vi "Do_Every_minute.vi"(1 "Ch Names":string[](array[string]), 2 "Values":dbl[](array[numeric]) format="%.2f") -> ()   [LabVIEW 2012]
uses:
  Do_Every_5mins.ctl
  Anemometry/Anemometry Sub Vis/Controls/In_Range.ctl
  ADAM Client/Sub VIs/ADAM Controls/Traverse_Level_State.ctl
  ADAM Client/Sub VIs/ADAM Controls/Valco_valve_ph.ctl
  ADAM_Global.vi
panel:
  in  "Disable Sending email to estates regarding Chilled water Temp":bool=TRUE
  in  "Max K Factor":dbl=2.7
  out "Case":T1
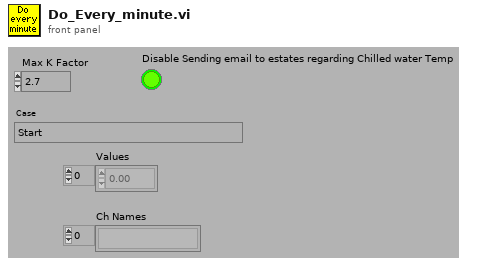
[diagram p1: front panel]
types:
  T1 = typedef "Do_Every_5mins.ctl" = enum16{"Start", "Update EnFlo Tunnel Speed Tweak", "Are EnFlo Tun Fan Bearings too Hot?", "Check EnFlo tweak factor?", "Are Inlet Screens Blocked?", "Tweak demanded chilled water temp", "Is Dew point meter Alive?", "Condensation Occurring", "Condensation Alert", "More checks", "Set FFID Valve to Measure", "End"}
  T2 = typedef "In_Range.ctl" = enum16{"%", "±", "% & ±"}
  T3 = typedef "Traverse_Level_State.ctl" = enum16{"Running", "Complete"}
  T4 = typedef "Client_State_Cluster.ctl" = cluster{"Client Name":string, "Traverse level State":T3, "People to Email":string[], "Next Contact Time":dbl}
  T5 = typedef "Valco_valve_ph.ctl" = u16
  T6 = cluster{"second":i32, "minute":i32, "hour":i32, "day of month":i32, "month":i32, "year":i32, "day of week":i32, "day of year":i32, "is DST":i32}
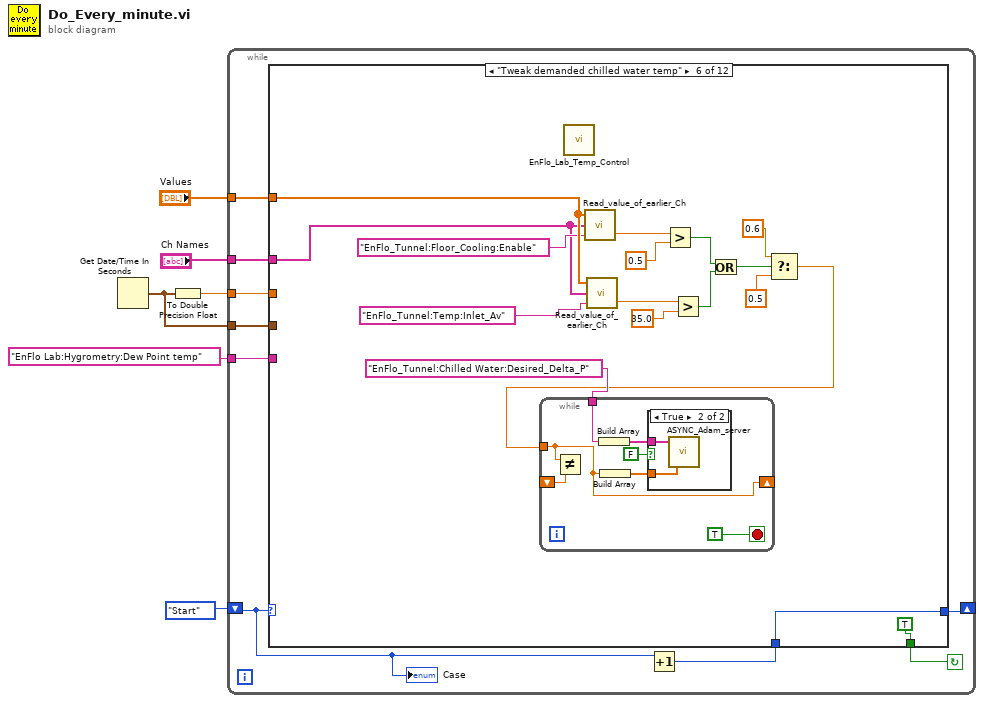
[diagram p0: block diagram]
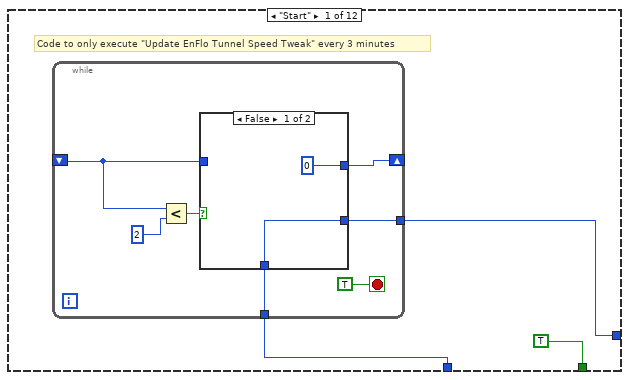
[diagram p2: hidden frame]
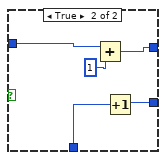
[diagram p3: hidden frame]
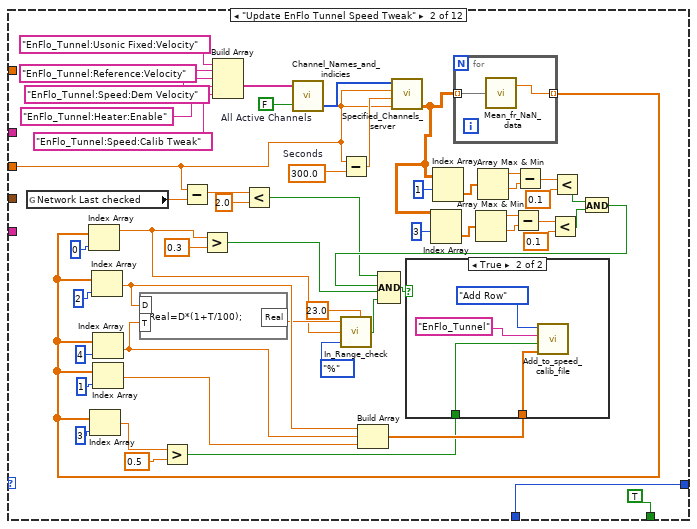
[diagram p4: hidden frame]
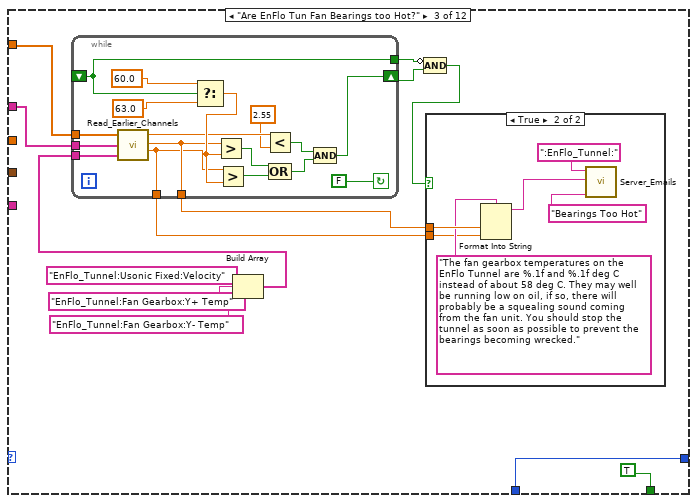
[diagram p6: hidden frame]
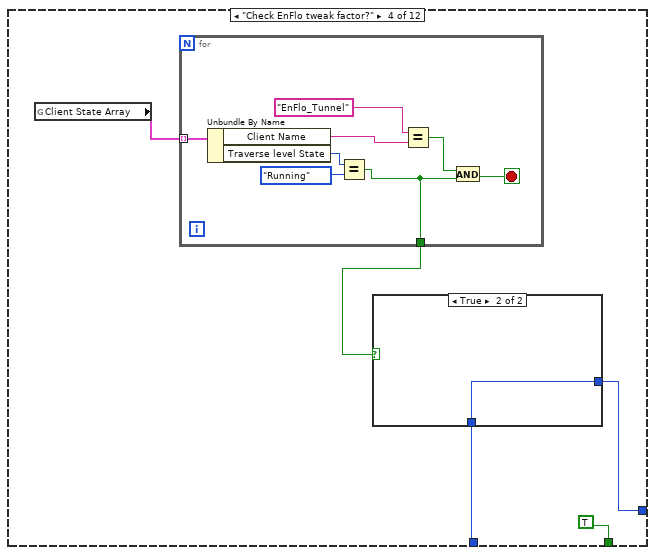
[diagram p8: hidden frame]
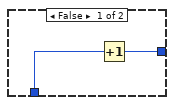
[diagram p9: hidden frame]
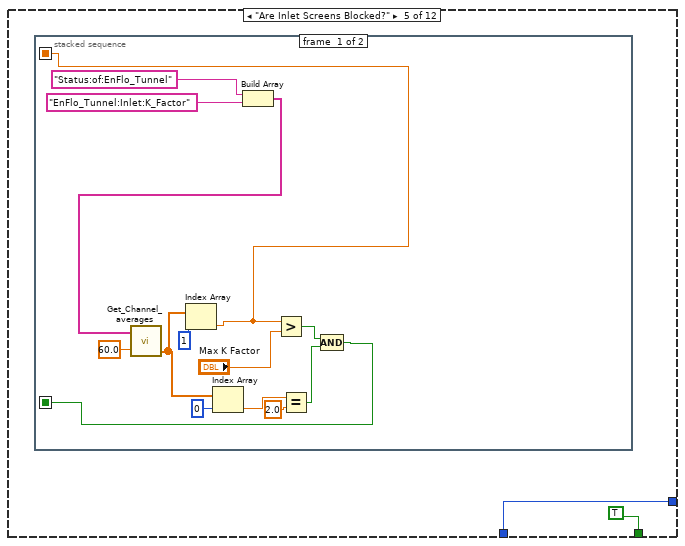
[diagram p10: hidden frame]
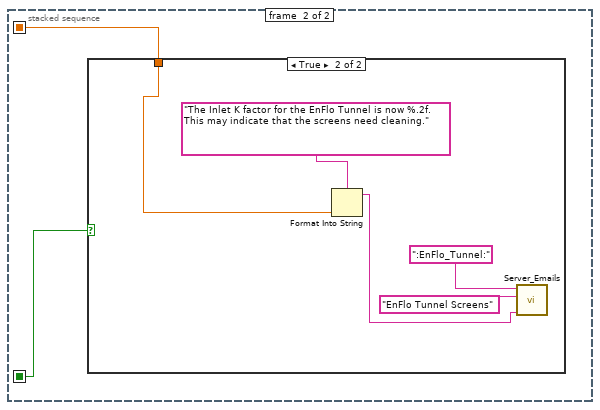
[diagram p11: hidden frame]
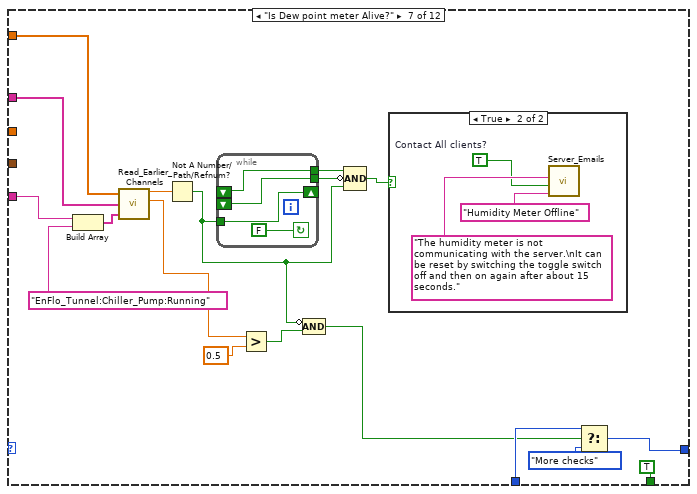
[diagram p14: hidden frame]
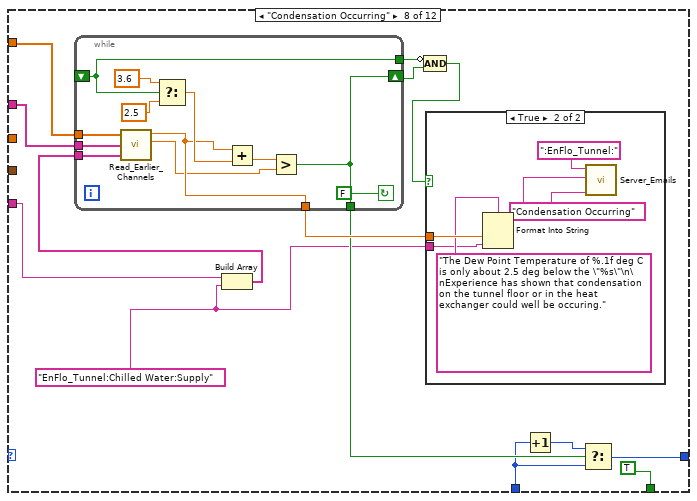
[diagram p16: hidden frame]
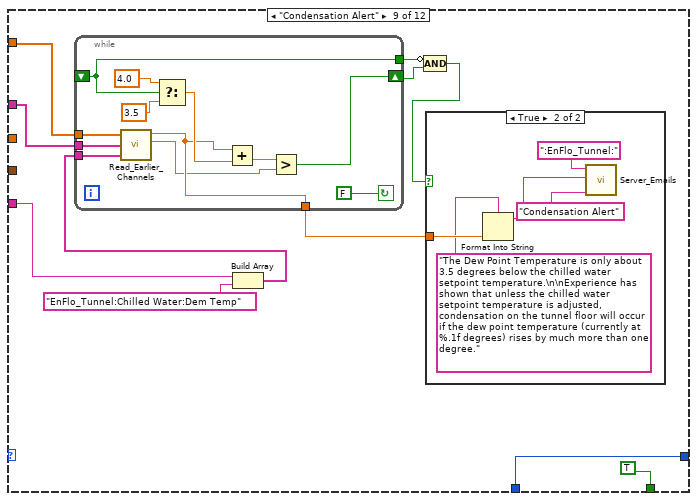
[diagram p18: hidden frame]
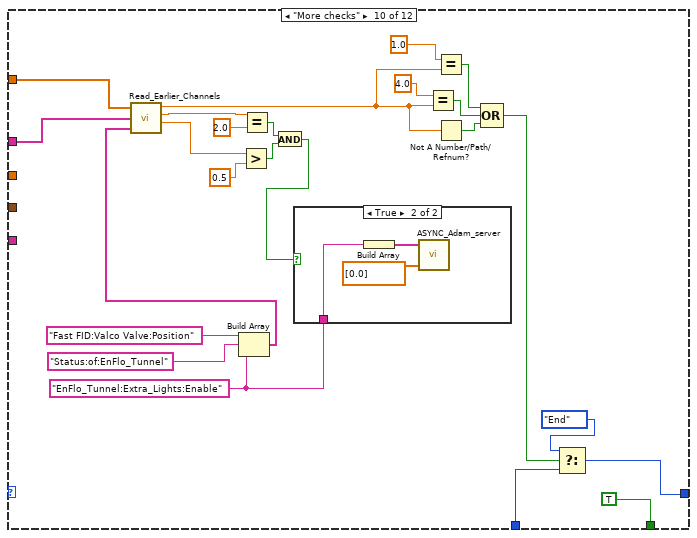
[diagram p20: hidden frame]
diagram:
  n1 = Get Date/Time In Seconds() -> (seconds since 1Jan1904=w1:timestamp)
  n2 = To Double Precision Float(number=w1) -> (double precision float=w2:dbl)
  n3 = while {
    tunnel: "EnFlo Lab:Hygrometry:Dew Point temp" -> [w9]
    tunnel: "Values" -> [w13]
    tunnel: "Ch Names" -> [w14]
    shift-left: Do_Every_5mins."Start" ("Case") -> [w10]
    shift-right: [w11] -> _
    tunnel: w2 -> [w8]
    tunnel: w1 -> [w7]
    stop <- w15 continue-if-true
    n4 = Increment(x=w10) -> (x+1=w12:T1)
    n5 = case shown="\"Tweak demanded chilled water temp\"" w10 {
      tunnel: [TRUE TRUE TRUE TRUE TRUE TRUE TRUE TRUE TRUE TRUE TRUE FALSE] -> w15
      tunnel: w14 -> [_ _ w102 _ _ w179 w207 w230 w257 w300 w307 w340]
      tunnel: w13 -> [_ _ w103 _ _ w181 w208 w231 w258 w301 w306 w339]
      tunnel: w12 -> [w16 w74 w93 w131 w145 w184 w199 w221 w260 w298 w325 w343]
      tunnel: [w17 w74 w93 w130 w145 w184 w211 w222 w260 w297 w325 w343] -> w11
      tunnel: w9 -> [_ _ _ _ _ _ w206 w224 w251 _ _ _]
      tunnel: w8 -> [_ w34 _ _ _ _ _ _ _ _ w324 _]
      tunnel: w7 -> [_ _ _ _ _ _ _ _ _ _ _ w341]
      frame "Start" {
        # "Code to only execute \"Update EnFlo Tunnel Speed Tweak\" every 3 minutes"
        n6 = while {
          shift-right: [w22] -> _
          shift-left: _ -> [w19]
          tunnel: [w21] -> w17
          tunnel: w16 -> [w20]
          stop <- TRUE stop-if-true
          n7 = Less?(x=w19, y=2) -> (x < y?=w23:bool)
          n8 = case shown="False" w23 {
            tunnel: [0 w30] -> w22
            tunnel: [w26 w28] -> w21
            tunnel: w20 -> [w26 w29]
            tunnel: w19 -> [_ w31]
            frame False {
            }
            frame True {
              n9 = Add(x=w31, y=1) -> (x+y=w30:i32)
              n10 = Increment(x=w29) -> (x+1=w28:T1)
            }
          }
        }
      }
      frame "Update EnFlo Tunnel Speed Tweak" {
        w68 = 300.0  # Seconds
        w70 = FALSE  # All Active Channels
        n11 = global read "ADAM_Global.vi" "Network Last checked"() -> (w35:dbl)
        n12 = Subtract(x=w34, y=w35) -> (x-y=w36:dbl)
        n13 = Build Array("EnFlo_Tunnel:Usonic Fixed:Velocity", "EnFlo_Tunnel:Reference:Velocity", "EnFlo_Tunnel:Speed:Dem Velocity", "EnFlo_Tunnel:Heater:Enable", "EnFlo_Tunnel:Speed:Calib Tweak") -> (w67:string[])
        n14 = Less?(x=w36, y=2.0) -> (x < y?=w33:bool)
        n15 = call "Channel_Names_and_indicies.vi"("All Active Channels"=w70, "Desired Ch Names"=w67) -> ("Indicies"=w69:i32[])  [unwired: 1 out]
        n16 = Subtract(x=w34, y=w68) -> (x-y=w66:dbl)
        n17 = call "Specified_Channels_server.vi"("End time"=w34, "Start time"=w66, "Clients time"=w34, "Requested channels"=w69) -> ("Output array"=w48:dbl[][])  [unwired: 1 in, 4 out]
        n18 = Index Array(array=w48, index (row)=3 ("Index")) -> (element=w50:dbl[])  [unwired: 1 in]
        n19 = Index Array(array=w48, index (row)=1 ("Index")) -> (element=w64:dbl[])  [unwired: 1 in]
        n20 = for {
          tunnel: w48 -> [w88] mode=indexing
          tunnel: [w87] -> w57 mode=indexing
          n21 = call "Mean_fr_NaN_data.vi"("Data"=w88) -> ("Mean value"=w87:dbl)  [unwired: 1 out]
        }
        n22 = Index Array(array=w57, index=0) -> (element=w41:dbl)
        n23 = Index Array(array=w57, index=3) -> (element=w77:dbl)
        n24 = Index Array(array=w57, index=2) -> (element=w43:dbl)
        n25 = Index Array(array=w57, index=4) -> (element=w44:dbl)
        n26 = Index Array(array=w57, index=1) -> (element=w55:dbl)
        n27 = formula code="Real=D*(1+T/100);"("D"=w43, "T"=w44) -> ("Real"=w42:dbl)
        n28 = Greater?(x=w77, y=0.5) -> (0:w56:bool)
        n29 = Greater?(x=w41, y=0.3) -> (0:w75:bool)
        n30 = call "In_Range_check.vi"("%"=23.0, "Mode"=In_Range."%", "Value"=w41, "Setpoint"=w42) -> ("In Range"=w38:bool)  [unwired: 1 in, 2 out]
        n31 = Build Array(w43, w44, w55) -> (w72:dbl[])
        n32 = Array Max & Min(array=w50) -> (max value=w51:dbl, min value=w52:dbl)  [unwired: 2 out]
        n33 = Array Max & Min(array=w64) -> (max value=w63:dbl, min value=w62:dbl)  [unwired: 2 out]
        n34 = Subtract(x=w51, y=w52) -> (x-y=w53:dbl)
        n35 = Subtract(x=w63, y=w62) -> (x-y=w61:dbl)
        n36 = Less?(x=w53, y=0.1) -> (x < y?=w47:bool)
        n37 = Less?(x=w61, y=0.1) -> (x < y?=w46:bool)
        n38 = And(x=w46, y=w47) -> (x .and. y?=w45:bool)
        n39 = Compound Arithmetic op=AND(w33, w45, w75, w38) -> (w71:bool)
        n40 = case shown="True" w71 {
          tunnel: w72 -> [_ w91]
          tunnel: w56 -> [_ w90]
          frame False {
          }
          frame True {
            n41 = call "Add_to_speed_calib_file.vi"("New Row"=w91, "Tunnel Heated?"=w90, "Rig Name"="EnFlo_Tunnel" ("y"), "Mode"=enum16{"Add Row", "Get Error Value"}."Add Row") -> ()  [unwired: 2 in, 2 out]
          }
        }
      }
      frame "Are EnFlo Tun Fan Bearings too Hot?" {
        n42 = Build Array("EnFlo_Tunnel:Usonic Fixed:Velocity", "EnFlo_Tunnel:Fan Gearbox:Y+ Temp", "EnFlo_Tunnel:Fan Gearbox:Y- Temp") -> (w101:string[])
        n43 = while {
          tunnel: [w107] -> w94
          tunnel: [w108] -> w95
          tunnel: [w117] -> w100
          shift-left: _ -> [w117]
          shift-right: [w109] -> w99
          tunnel: w101 -> [w120]
          tunnel: w102 -> [w121]
          tunnel: w103 -> [w122]
          stop <- FALSE continue-if-true
          n44 = call "Read_Earlier_Channels.vi"("Present scan array"=w122, "Ch names"=w121, "Desired Channels"=w120) -> ("Index 0"=w115:dbl, "Index 1"=w108:dbl, "Index 2"=w107:dbl)  [unwired: 3 out]
          n45 = Select(t=60.0, s=w117, f=63.0) -> (s? t:f=w116:dbl)
          n46 = Greater?(x=w108, y=w116) -> (0:w113:bool)
          n47 = Greater?(x=w107, y=w116) -> (0:w112:bool)
          n48 = Less?(x=w115, y=2.55) -> (x < y?=w111:bool)
          n49 = Compound Arithmetic op=OR(w113, w112) -> (w110:bool)
          n50 = Compound Arithmetic op=AND(w111, w110) -> (w109:bool)
        }
        n51 = Compound Arithmetic op=AND(invert w100, w99) -> (w98:bool)
        n52 = case shown="True" w98 {
          tunnel: w95 -> [_ w126]
          tunnel: w94 -> [_ w123]
          frame False {
          }
          frame True {
            n53 = Format Into String(format string="The fan gearbox temperatures on the EnFlo Tunnel are %.1f and %.1f deg C instead of about 58 deg C. They may well be running low on oil, if so, there will probably be a squealing sound coming from the fan unit. You should stop the tunnel as soon as possible to prevent the bearings becoming wrecked." ("Format String"), w126, w123) -> (resulting string=w125:string)  [unwired: 2 in, 1 out]
            n54 = call "Server_Emails.vi"("Client Name Contains"=":EnFlo_Tunnel:", "Message"=w125, "Subject"="Bearings Too Hot" ("Error Type")) -> ()  [unwired: 2 in, 3 out]
          }
        }
      }
      frame "Check EnFlo tweak factor?" {
        n55 = global read "ADAM_Global.vi" "Client State Array"() -> (w132:T4[])
        n56 = for {
          tunnel: w132 -> [w144] mode=indexing
          tunnel: [w137] -> w129
          stop <- w138 stop-if-true
          n57 = Unbundle By Name(w144) -> ("Client Name"=w140:string, "Traverse level State"=w143:T3)
          n58 = Equal?(x=w143, y=Traverse_Level_State."Running" ("Traverse level State")) -> (x = y?=w137:bool)
          n59 = Equal?(x="EnFlo_Tunnel" ("y"), y=w140) -> (x = y?=w139:bool)
          n60 = And(x=w139, y=w137) -> (x .and. y?=w138:bool)
        }
        n61 = case shown="True" w129 {
          tunnel: w131 -> [w135 w136]
          tunnel: [w134 w136] -> w130
          frame False {
            n62 = Increment(x=w135) -> (x+1=w134:T1)
          }
          frame True {
          }
        }
      }
      frame "Are Inlet Screens Blocked?" {
        n63 = stacked-sequence {
          seq-local: [w147 _] -> [_ w162]
          seq-local: [w150 _] -> [_ w161]
          frame #0 {
            n64 = Build Array("Status:of:EnFlo_Tunnel", "EnFlo_Tunnel:Inlet:K_Factor") -> (w152:string[])
            n65 = call "Get_Channel_averages.vi"("Desired Ch Names"=w152, "Averaging time (mins)"=60.0) -> ("number"=w158:dbl[])  [unwired: 1 in, 2 out]
            n66 = Index Array(array=w158, index=1) -> (element=w147:dbl)
            n67 = Index Array(array=w158, index=0) -> (element=w157:dbl)
            n68 = Greater?(x=w147, y="Max K Factor") -> (0:w149:bool)
            n69 = Equal?(x=w157, y=2.0) -> (x = y?=w155:bool)
            n70 = Compound Arithmetic op=AND(w149, w155) -> (w150:bool)
          }
          frame #1 {
            n71 = case shown="True" w161 {
              tunnel: w162 -> [_ w166]
              frame False {
              }
              frame True {
                n72 = Format Into String(format string="The Inlet K factor for the EnFlo Tunnel is now %.2f. This may indicate that the screens need cleaning." ("Format String"), w166) -> (resulting string=w164:string)  [unwired: 2 in, 1 out]
                n73 = call "Server_Emails.vi"("Client Name Contains"=":EnFlo_Tunnel:", "Message"="EnFlo Tunnel Screens", "Subject"=w164) -> ()  [unwired: 2 in, 3 out]
              }
            }
          }
        }
      }
      frame "Tweak demanded chilled water temp" {
        n74 = call "EnFlo_Lab_Temp_Control.vi"() -> ()  [unwired: 1 out]
        n75 = call "Read_value_of_earlier_Ch.vi"("Desired Ch to Read"="EnFlo_Tunnel:Floor_Cooling:Enable", "Ch names"=w179, "Present scan array"=w181) -> ("Value"=w177:dbl)  [unwired: 1 in, 1 out]
        n76 = call "Read_value_of_earlier_Ch.vi"("Desired Ch to Read"="EnFlo_Tunnel:Temp:Inlet_Av", "Ch names"=w179, "Present scan array"=w181) -> ("Value"=w175:dbl)  [unwired: 1 in, 1 out]
        n77 = Greater?(x=w177, y=0.5) -> (0:w173:bool)
        n78 = Greater?(x=w175, y=35.0) -> (0:w172:bool)
        n79 = Or(x=w173, y=w172) -> (x .or. y?=w171:bool)
        n80 = Select(t=0.6, s=w171, f=0.5 ("t")) -> (s? t:f=w168:dbl)
        n81 = while {
          shift-right: [w187] -> _
          shift-left: _ -> [w188]
          tunnel: w168 -> [w187]
          tunnel: "EnFlo_Tunnel:Chilled Water:Desired_Delta_P" -> [w189]
          stop <- TRUE stop-if-true
          n82 = Not Equal?(x=w187, y=w188) -> ()  [unwired: 1 out]
          n83 = Build Array(w189) -> (w190:string[])
          n84 = Build Array(w187) -> (w191:dbl[])
          n85 = case shown="True" FALSE {
            tunnel: w191 -> [_ w193]
            tunnel: w190 -> [_ w192]
            frame False {
            }
            frame True {
              n86 = call "ASYNC_Adam_server.vi"("Values"=w193, "Channel Names"=w192) -> ()  [unwired: 1 in, 3 out]
            }
          }
        }
      }
      frame "Is Dew point meter Alive?" {
        n87 = Build Array(w206, "EnFlo_Tunnel:Chiller_Pump:Running") -> (w204:string[])
        n88 = call "Read_Earlier_Channels.vi"("Present scan array"=w208, "Ch names"=w207, "Desired Channels"=w204) -> ("Index 0"=w203:dbl, "Index 1"=w201:dbl)  [unwired: 4 out]
        n89 = Not A Number/Path/Refnum?(number/path/refnum=w203) -> (NaN/Path/Refnum?=w196:bool)
        n90 = while {
          tunnel: [w213] -> w194
          tunnel: [w214] -> w195
          shift-left: _ -> [w214]
          tunnel: w196 -> [w215]
          shift-left: _ -> [w213]
          shift-right: [w215] -> _
          stop <- FALSE continue-if-true
        }
        n91 = Greater?(x=w201, y=0.5) -> (0:w200:bool)
        n92 = Compound Arithmetic op=AND(invert w196, w200) -> (w197:bool)
        n93 = Compound Arithmetic op=AND(w194, invert w195, w196) -> (w209:bool)
        n94 = case shown="True" w209 {
          frame False {
          }
          frame True {
            w216 = TRUE  # Contact All clients?
            n95 = call "Server_Emails.vi"("Message"="The humidity meter is not communicating with the server.\nIt can be reset by switching the toggle switch off and then on again after about 15 seconds." ("Bundle Element"), "Contact All clients?"=w216, "Subject"="Humidity Meter Offline" ("Error Type")) -> ()  [unwired: 2 in, 3 out]
          }
        }
        n96 = Select(t=w199, s=w197, f=Do_Every_5mins."More checks" ("Case")) -> (s? t:f=w211:T1)
      }
      frame "Condensation Occurring" {
        w219 = "EnFlo_Tunnel:Chilled Water:Supply"
        n97 = Build Array(w224, w219) -> (w229:string[])
        n98 = while {
          tunnel: [w234] -> w223
          tunnel: [w236] -> w225
          tunnel: [w237] -> w228
          shift-left: _ -> [w237]
          shift-right: [w234] -> w227
          tunnel: w229 -> [w242]
          tunnel: w230 -> [w243]
          tunnel: w231 -> [w244]
          stop <- FALSE continue-if-true
          n99 = call "Read_Earlier_Channels.vi"("Present scan array"=w244, "Ch names"=w243, "Desired Channels"=w242) -> ("Index 0"=w236:dbl, "Index 1"=w235:dbl)  [unwired: 4 out]
          n100 = Select(t=3.6, s=w237, f=2.5) -> (s? t:f=w238:dbl)
          n101 = Add(x=w236, y=w238) -> (x+y=w241:dbl)
          n102 = Greater?(x=w241, y=w235) -> (0:w234:bool)
        }
        n103 = Compound Arithmetic op=AND(invert w228, w227) -> (w226:bool)
        n104 = case shown="True" w226 {
          tunnel: w225 -> [_ w248]
          tunnel: w219 -> [_ w245]
          frame False {
          }
          frame True {
            n105 = Format Into String(format string="The Dew Point Temperature of %.1f deg C is only about 2.5 deg below the \"%s\"\n\nExperience has shown that condensation on the tunnel floor or in the heat exchanger could well be occuring." ("Format String"), w248, w245) -> (resulting string=w247:string)  [unwired: 2 in, 1 out]
            n106 = call "Server_Emails.vi"("Client Name Contains"=":EnFlo_Tunnel:", "Message"=w247, "Subject"="Condensation Occurring" ("Error Type")) -> ()  [unwired: 2 in, 3 out]
          }
        }
        n107 = Increment(x=w221) -> (x+1=w220:T1)
        n108 = Select(t=w220, s=w223, f=w221) -> (s? t:f=w222:T1)
      }
      frame "Condensation Alert" {
        n109 = Build Array(w251, "EnFlo_Tunnel:Chilled Water:Dem Temp") -> (w256:string[])
        n110 = while {
          tunnel: [w264] -> w252
          tunnel: [w266] -> w255
          shift-left: _ -> [w266]
          shift-right: [w265] -> w254
          tunnel: w256 -> [w271]
          tunnel: w257 -> [w272]
          tunnel: w258 -> [w273]
          stop <- FALSE continue-if-true
          n111 = call "Read_Earlier_Channels.vi"("Present scan array"=w273, "Ch names"=w272, "Desired Channels"=w271) -> ("Index 0"=w264:dbl, "Index 1"=w263:dbl)  [unwired: 4 out]
          n112 = Select(t=4.0, s=w266, f=3.5) -> (s? t:f=w267:dbl)
          n113 = Add(x=w264, y=w267) -> (x+y=w270:dbl)
          n114 = Greater?(x=w270, y=w263) -> (0:w265:bool)
        }
        n115 = Compound Arithmetic op=AND(invert w255, w254) -> (w253:bool)
        n116 = case shown="True" w253 {
          tunnel: w252 -> [_ w276]
          frame False {
          }
          frame True {
            n117 = Format Into String(format string="The Dew Point Temperature is only about 3.5 degrees below the chilled water setpoint temperature.\n\nExperience has shown that unless the chilled water setpoint temperature is adjusted, condensation on the tunnel floor will occur if the dew point temperature (currently at %.1f degrees) rises by much more than one degree." ("Format String"), w276) -> (resulting string=w275:string)  [unwired: 2 in, 1 out]
            n118 = call "Server_Emails.vi"("Client Name Contains"=":EnFlo_Tunnel:", "Message"=w275, "Subject"="Condensation Alert" ("Error Type")) -> ()  [unwired: 2 in, 3 out]
          }
        }
      }
      frame "More checks" {
        w280 = "EnFlo_Tunnel:Extra_Lights:Enable"
        n119 = Build Array("Fast FID:Valco Valve:Position", "Status:of:EnFlo_Tunnel", w280) -> (w295:string[])
        n120 = call "Read_Earlier_Channels.vi"("Present scan array"=w301, "Ch names"=w300, "Desired Channels"=w295) -> ("Index 0"=w288:dbl, "Index 1"=w286:dbl, "Index 2"=w284:dbl)  [unwired: 3 out]
        n121 = Greater?(x=w284, y=0.5) -> (0:w282:bool)
        n122 = Equal?(x=w286, y=2.0) -> (x = y?=w281:bool)
        n123 = And(x=w281, y=w282) -> (x .and. y?=w279:bool)
        n124 = case shown="True" w279 {
          tunnel: w280 -> [_ w305]
          frame False {
          }
          frame True {
            n125 = Build Array(w305) -> (w304:string[])
            n126 = call "ASYNC_Adam_server.vi"("Values"=dbl[] [0.0], "Channel Names"=w304) -> ()  [unwired: 1 in, 3 out]
          }
        }
        n127 = Equal?(x=4.0, y=w288) -> (x = y?=w292:bool)
        n128 = Equal?(x=1.0, y=w288) -> (x = y?=w291:bool)
        n129 = Not A Number/Path/Refnum?(number/path/refnum=w288) -> (NaN/Path/Refnum?=w293:bool)
        n130 = Compound Arithmetic op=OR(w291, w292, w293) -> (w290:bool)
        n131 = Select(t=Do_Every_5mins."End" ("Case"), s=w290, f=w298) -> (s? t:f=w297:T1)
      }
      frame "Set FFID Valve to Measure" {
        w323 = FALSE  # All Active Channels
        n132 = Build Array("Fast FID:Valco Valve:Position") -> (w321:string[])
        n133 = call "Channel_Names_and_indicies.vi"("All Active Channels"=w323, "Desired Ch Names"=w321) -> ("Indicies"=w322:i32[])  [unwired: 1 out]
        n134 = Subtract(x=w324, y=700.0) -> (x-y=w319:dbl)
        n135 = call "Specified_Channels_server.vi"("End time"=w324, "Start time"=w319, "Clients time"=w324, "Requested channels"=w322) -> ("Output array"=w316:dbl[][])  [unwired: 1 in, 4 out]
        n136 = Index Array(array=w316, index (row)=0 ("Index")) -> (element=w312:dbl[])  [unwired: 1 in]
        n137 = Not A Number/Path/Refnum?(number/path/refnum=w312) -> (NaN/Path/Refnum?=w311:bool[])
        n138 = Or Array Elements(Boolean array=w311) -> (logical OR=w309:bool)
        n139 = Array Max & Min(array=w312) -> (max value=w314:dbl, min value=w315:dbl)  [unwired: 2 out]
        n140 = Subtract(x=w314, y=w315) -> (x-y=w313:dbl)
        n141 = Equal To 0?(x=w313) -> (x = 0?=w310:bool)
        n142 = Compound Arithmetic op=AND(w310, invert w309) -> (w308:bool)
        n143 = case shown="True" w308 {
          tunnel: w307 -> [_ w333]
          tunnel: w306 -> [_ w332]
          frame False {
          }
          frame True {
            n144 = Build Array("FFID:System:Enable") -> (w330:string[])
            n145 = call "Read_Earlier_Channels.vi"("Present scan array"=w332, "Ch names"=w333, "Desired Channels"=w330) -> ("Index 0"=w329:dbl)  [unwired: 5 out]
            n146 = Greater?(x=w329, y=0.5) -> (0:w327:bool)
            n147 = case shown="True" w327 {
              frame False {
                n148 = Build Array(0.0) -> (w335:dbl[])
                n149 = Build Array("GMU:Gas:Enable") -> (w337:string[])
                n150 = call "ASYNC_Adam_client.vi"("Values"=w335, "Channel Names"=w337) -> ()  [unwired: 2 out]
              }
              frame True {
                w338 = T5 4 items=["", "Zero Air", "Calib 1", "Calib 2", "Measure"] ("Requested Position")
                n151 = call "Fast_FID_Valve_Control.vi"("Requested Position"=w338) -> ()  [unwired: 7 out]
              }
            }
          }
        }
      }
      frame "End" {
        n152 = stacked-sequence {
          seq-local: [w350 _] -> [_ w370]
          seq-local: [w344 _] -> [_ w367]
          tunnel: w341 -> [w355 _]
          tunnel: w340 -> [w347 w369]
          tunnel: w339 -> [w348 w368]
          frame #0 {
            n153 = call <vilib>:"LV70TimeStampToDateRec.vi"("time stamp"=w355) -> ("date time rec"=w356:T6)
            n154 = Unbundle By Name(w356) -> ("hour"=w354:i32, "day of week"=w353:i32)
            n155 = while {
              tunnel: w354 -> [w366]
              tunnel: w353 -> [w364]
              shift-right: [w359] -> w351
              shift-left: _ -> [w358]
              tunnel: [w358] -> w352
              stop <- FALSE continue-if-true
              n156 = Equal?(x=w366, y=10) -> (x = y?=w360:bool)
              n157 = In Range and Coerce(upper limit=7, x=w364, lower limit=1) -> (In Range?=w361:bool)  [unwired: 1 out]
              n158 = And(x=w360, y=w361) -> (x .and. y?=w359:bool)
            }
            n159 = call "Read_value_of_earlier_Ch.vi"("Desired Ch to Read"="Uni:Chilled Water:Temp", "Ch names"=w347, "Present scan array"=w348) -> ("Value"=w344:dbl)  [unwired: 1 in, 1 out]
            n160 = Greater?(x=w344, y=15.0) -> (0:w345:bool)
            n161 = Compound Arithmetic op=AND(w345, invert w352, w351) -> (w350:bool)
          }
          frame #1 {
            n162 = case shown="True" w370 {
              tunnel: w369 -> [_ _]
              tunnel: w368 -> [_ _]
              tunnel: w367 -> [_ w378]
              frame False {
              }
              frame True {
                n163 = Select(t=string[] [], s="Disable Sending email to estates regarding Chilled water Temp", f=string[] ["efmenquiries@surrey.ac.uk"] ("Extra People to Email")) -> (s? t:f=w371:string[])
                n164 = Format Into String(format string="Dear Estates\n\nThe monitoring system in the EnFlo Lab (01AB01) is currently indicating that the Chilled water in the AB Building is at %d deg C.\n\nPlease could you arrange for somebody to come and investigate this please.\n\nThanks very much\n\nPaul Hayden x9545  or Mobile  07961 608409", w378) -> (resulting string=w377:string)  [unwired: 2 in, 1 out]
                n165 = call "Server_Emails.vi"("Message"=w377, "Contact All clients?"=TRUE, "Subject"="Chilled water in AB Building above 15 deg C" ("Error Type"), "Extra People to Email"=w371) -> ()  [unwired: 1 in, 3 out]
              }
            }
          }
        }
      }
    }
    "Case" <- w10
  }
